vi "StartStopACQ.vi"(8 "error in (no error)":errorcluster, 10 "Start Stop":bool, 11 "GUI Actor in":refnum<class "GUI Actor.lvclass">) -> (0 "error out":errorcluster, 3 "GUI Actor out":refnum<class "GUI Actor.lvclass">)   [LabVIEW 2019, in "GUI Actor.lvlib" / "GUI Actor.lvclass"]
uses:
  GUI Actor.lvclass
  GUI Actor.lvclass/GUI Actor.ctl
  Measurment Actor/Measurment Actor Messages/Start Stop grpagh Msg/Start Stop grpagh Msg.lvclass/Start Stop grpagh Msg.ctl
  <vilib>/ActorFramework/Message Enqueuer/Message Enqueuer.lvclass/Message Enqueuer.ctl
  <vilib>/ActorFramework/Message Enqueuer/Enqueue.vi
  Measurment Actor/Measurment Actor Messages/Start Stop grpagh Msg/Start Stop grpagh Msg.lvclass
  C:/Program Files (x86)/National Instruments/LabVIEW 2019/vi.lib/ActorFramework/Message/Message.lvclass
  <vilib>/ActorFramework/Message Priority Queue/Priority Enqueue.vi
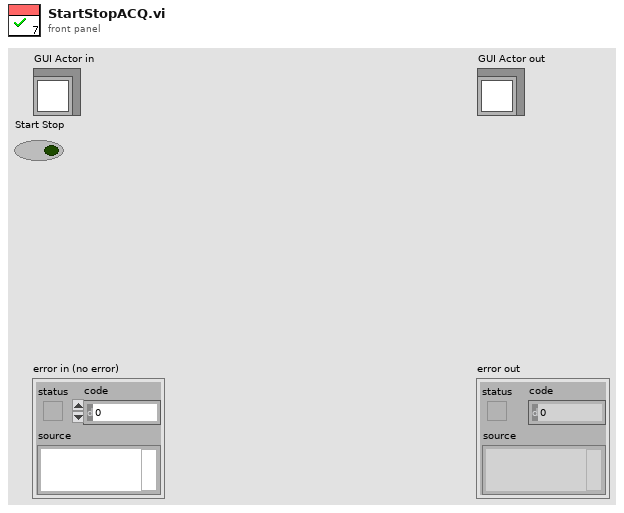
[diagram p1: front panel]
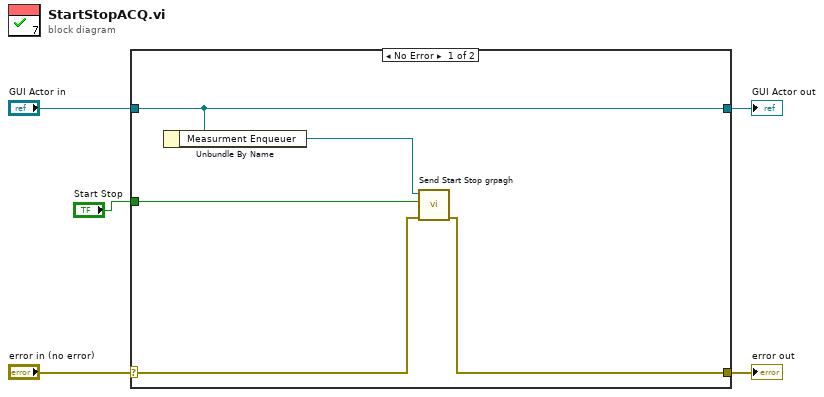
[diagram p0: block diagram]
diagram:
  n1 = case shown="No Error" "error in (no error)" {
    selector: "error in (no error)" -> [w8 w12]
    tunnel: [w7 w12] -> w4
    tunnel: [w10 w11] -> w2
    tunnel: "GUI Actor in" -> [w10 w11]
    tunnel: "Start Stop" -> [w6 _]
    frame No Error {
      n2 = Unbundle By Name(w10) -> ("Measurment Enqueuer"=w9:refnum<class "Message Enqueuer.lvclass">)
      n3 = call "Send Start Stop grpagh.vi"("error in (no error)"=w8, "Start Stop"=w6, "Message Enqueuer"=w9) -> ("error out"=w7:errorcluster)  [unwired: 7 in, 1 out]
    }
    frame Error {
    }
  }
  "error out" <- w4
  "GUI Actor out" <- w2
